vi "update setpoint.vi"(7 "exp exec in":T1={"data file"={"autosave"=FALSE, "File refnum"=refnum, "data file path"=path ""}, "T log file"={"File refnum"=refnum, "T log file path"=path "", "exists"=FALSE}, "exp seq"={"wave params"={"Num of avg"=0, "Num points"=1000, "Meas rate (Hz)"=100000.0}, "Setpoints"=[], "#"=-1, "index"=-1, "elapsed time (s)"=0.0, "set time (s)"=0.0, "min settle (s)"=30.0, " Exec Status"=enum."Settling"}, "error"={"status"=FALSE, "code"=0, "source"=""}}) -> (2 "Num set points":i32, 3 "current setpoint index":i32, 4 "current set point":dbl, 8 "exp exec out":T1={"data file"={"autosave"=FALSE, "File refnum"=refnum, "data file path"=path ""}, "T log file"={"File refnum"=refnum, "T log file path"=path "", "exists"=FALSE}, "exp seq"={"wave params"={"Num of avg"=0, "Num points"=1000, "Meas rate (Hz)"=100000.0}, "Setpoints"=[], "#"=-1, "index"=-1, "elapsed time (s)"=0.0, "set time (s)"=0.0, "min settle (s)"=30.0, " Exec Status"=enum."Settling"}, "error"={"status"=FALSE, "code"=0, "source"=""}}, 15 "Setpoints":dbl[](array[numeric]))   [LabVIEW 2019]
doc: "This is a Bug C(T) subVI.\n\nThis subVI updates the setpoint, meas status, and the bug global variables from the executive thread.\n\nPaul K Dixon\nP3600\nCSUSB Physics"
uses:
  typedefs/PID exec cluster.ctl
  typedefs/data file info.ctl
  typedefs/bug temp file info.ctl
  typedefs/exp seq cluster.ctl
  typedefs/wvfm acq params.ctl
  typedefs/bug meas status.ctl
  typedefs/temp mode enum.ctl
  globals/Bug globals.vi
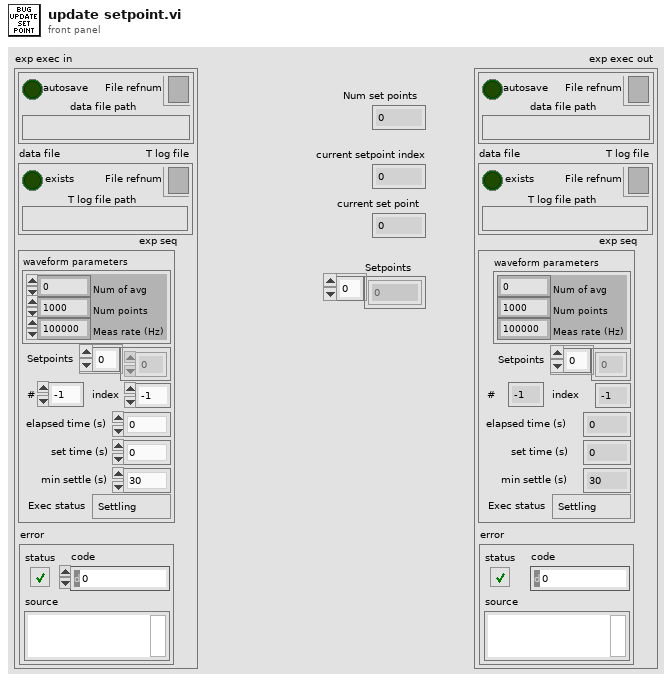
[diagram p1: front panel]
types:
  T1 = typedef "PID exec cluster.ctl" = cluster{"data file":T2, "T log file":T3, "exp seq":T4, "error":errorcluster}
  T2 = typedef "data file info.ctl" = cluster{"autosave":bool, "File refnum":refnum<file>, "data file path":path}
  T3 = typedef "bug temp file info.ctl" = cluster{"File refnum":refnum<file>, "T log file path":path, "exists":bool}
  T4 = typedef "exp seq cluster.ctl" = cluster{"wave params":T5, "Setpoints":dbl[], "#":i32, "index":i32, "elapsed time (s)":dbl, "set time (s)":dbl, "min settle (s)":dbl, " Exec Status":T6}
  T5 = typedef "wvfm acq params.ctl" = cluster{"Num of avg":i32, "Num points":i32, "Meas rate (Hz)":dbl}
  T6 = typedef "bug meas status.ctl" = enum32{"Settling", "Measuring", "Holding", "Exit"}
  T7 = typedef "temp cont cluster.ctl" = cluster{"T exec":T8, "T status":T10, "T params":T12, "utility":T13}
  T8 = typedef "temp exec cluster.ctl" = cluster{"T mode":T9, "exec setpoint":dbl, "reset":bool, "man power":dbl, "man":bool, "log":bool, "clear":bool}
  T9 = typedef "temp mode enum.ctl" = enum16{"settling", "measuring", "holding", "Exit"}
  T10 = typedef "temp indicator.ctl" = cluster{"Control status":T11, "Temp":dbl, "Power":dbl, "Time in settle band":dbl, "Settled":bool, "Low":bool, "High":bool, "Setpoint":dbl, "Control":bool, "In Settle Band":bool}
  T11 = typedef "temp control status.ctl" = enum16{"In Settle Band", "In Control Band", "Below Control Band", "Above Control Band"}
  T12 = typedef "PID control parameters.ctl" = cluster{"Setpoint":dbl, "Control Bandwidth":dbl, "Integral Time":dbl, "Int\nON":bool, "Derivative Tme":dbl, "Der\nON":bool, "Settle Bandwidth":dbl, "Settle Time":dbl}
  T13 = typedef "temp cont utility.ctl" = cluster{"meas index":i32, "wait (ms)":i32, "H Vmax":dbl, "power out":dbl, "heat volt out":dbl, "heat volt in":dbl, "therm volt":dbl, "t T P hist":dbl[][], "cont hist":dbl[][]}
  T14 = typedef "measurement.ctl" = cluster{"wvfm params":T5, "avg":waveform(dbl), "raw wvfms":waveform(dbl)[], "progress":cluster{"avg done":bool, "meas index":i32, "N waves":i32}, "t (s)":dbl}
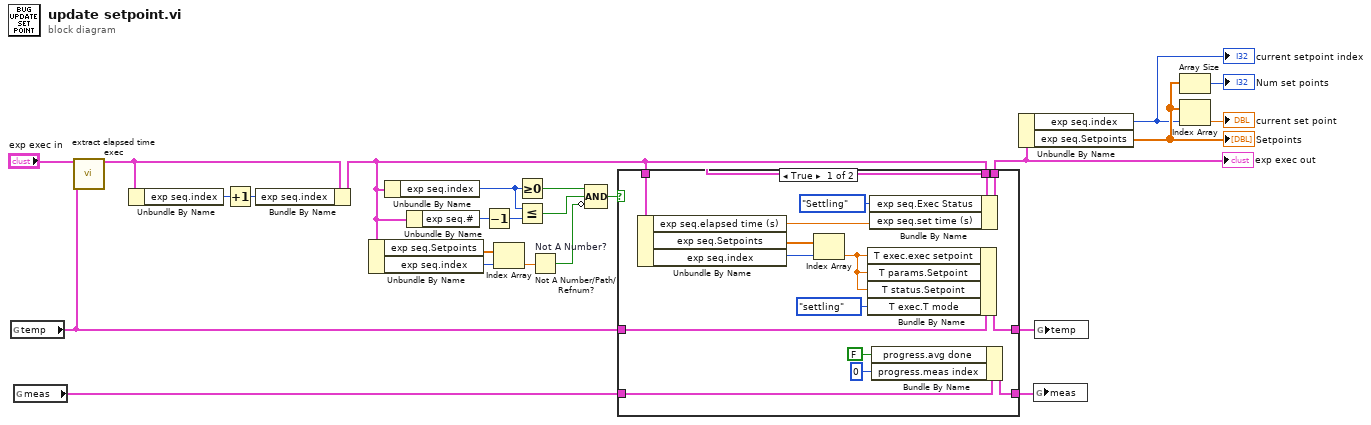
[diagram p0: block diagram]
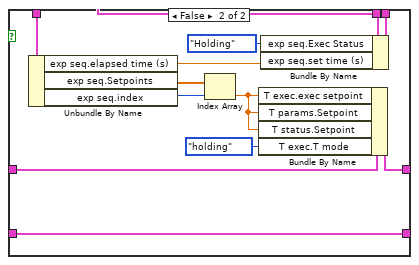
[diagram p2: hidden frame]
diagram:
  n1 = global read "Bug globals.vi" "temp"() -> (w13:T7)
  n2 = global read "Bug globals.vi" "meas"() -> (w2:T14)
  n3 = call "extract elapsed time exec.vi"("exp exec"="exp exec in", "temp"=w13) -> ("exec out"=w14:T1)  [unwired: 12 in, 1 out]
  n4 = Unbundle By Name(w14) -> ("exp seq.index"=w23:i32)
  n5 = Increment(x=w23) -> (x+1=w22:i32)
  n6 = Bundle By Name(cluster=w14, "exp seq.index"=w22) -> (w6:T1)
  n7 = Unbundle By Name(w6) -> ("exp seq.Setpoints"=w7:dbl[], "exp seq.index"=w8:i32)
  n8 = Unbundle By Name(w6) -> ("exp seq.index"=w19:i32)
  n9 = Unbundle By Name(w6) -> ("exp seq.#"=w21:i32)
  n10 = Decrement(x=w21) -> (x-1=w20:i32)
  n11 = Index Array(array=w7, index=w8) -> (element=w5:dbl)
  n12 = Greater Or Equal To 0?(x=w19) -> (x >= 0?=w18:bool)
  n13 = Less Or Equal?(x=w19, y=w20) -> (x <= y?=w17:bool)
  n14 = Not A Number/Path/Refnum? "Not A Number?"(number/path/refnum=w5) -> (NaN/Path/Refnum?=w4:bool)
  n15 = Compound Arithmetic op=AND(w18, w17, invert w4) -> (w16:bool)
  n16 = case shown="True" w16 {
    tunnel: [w39 w51] -> w24
    tunnel: [w37 w49] -> w12
    tunnel: w6 -> [w35 w47]
    tunnel: w13 -> [w33 w45]
    tunnel: w6 -> [w31 w43]
    tunnel: w2 -> [w28 w40]
    tunnel: [w27 w40] -> w1
    frame True {
      n17 = Unbundle By Name(w31) -> ("exp seq.elapsed time (s)"=w29:dbl, "exp seq.Setpoints"=w38:dbl[], "exp seq.index"=w34:i32)
      n18 = Index Array(array=w38, index=w34) -> (element=w36:dbl)
      n19 = Bundle By Name(cluster=w33, "T exec.exec setpoint"=w36, "T params.Setpoint"=w36, "T status.Setpoint"=w36, "T exec.T mode"=temp_mode_enum."settling") -> (w39:T7)
      n20 = Bundle By Name(cluster=w35, "exp seq.Exec Status"=bug_meas_status."Settling" ("exp seq. Exec Status"), "exp seq.set time (s)"=w29) -> (w37:T1)
      n21 = Bundle By Name(cluster=w28, "progress.avg done"=FALSE, "progress.meas index"=0) -> (w27:T14)
    }
    frame False {
      n22 = Unbundle By Name(w43) -> ("exp seq.elapsed time (s)"=w41:dbl, "exp seq.Setpoints"=w50:dbl[], "exp seq.index"=w46:i32)
      n23 = Index Array(array=w50, index=w46) -> (element=w48:dbl)
      n24 = Bundle By Name(cluster=w45, "T exec.exec setpoint"=w48, "T params.Setpoint"=w48, "T status.Setpoint"=w48, "T exec.T mode"=temp_mode_enum."holding") -> (w51:T7)
      n25 = Bundle By Name(cluster=w47, "exp seq.Exec Status"=bug_meas_status."Holding" ("exp seq. Exec Status"), "exp seq.set time (s)"=w41) -> (w49:T1)
    }
  }
  "exp exec out" <- w12
  n26 = Unbundle By Name(w12) -> ("exp seq.index"=w3:i32, "exp seq.Setpoints"=w10:dbl[])
  "Setpoints" <- w10
  "current setpoint index" <- w3
  n27 = global write "Bug globals.vi" "meas"(w1) -> ()
  n28 = global write "Bug globals.vi" "temp"(w24) -> ()
  n29 = Array Size(array=w10) -> (size(s)=→"Num set points":i32)
  n30 = Index Array(array=w10, index=w3) -> (element=→"current set point":dbl)
